vi "find_fish_position.vi"() -> ()   [LabVIEW 2012]
uses:
  labview/find_fish_position.lvlib
  bin/find_fish_position.dll
panel:
  in  "shift":i32=10
  in  "ROI height":i32=256
  in  "ROI width":i32=256
  in  "setROI":bool
  in  "Esize (open)":i32(slide)=4 scale=3.0..10.0
  out "Centroid":cluster{"y":i32, "x":i32}
  out "Image":T1(plugin-control)
  in  "Esize (close)":i32(slide)=4 scale=3.0..10.0
  in  "Threshold":i32(slide)=205 scale=50.0..255.0
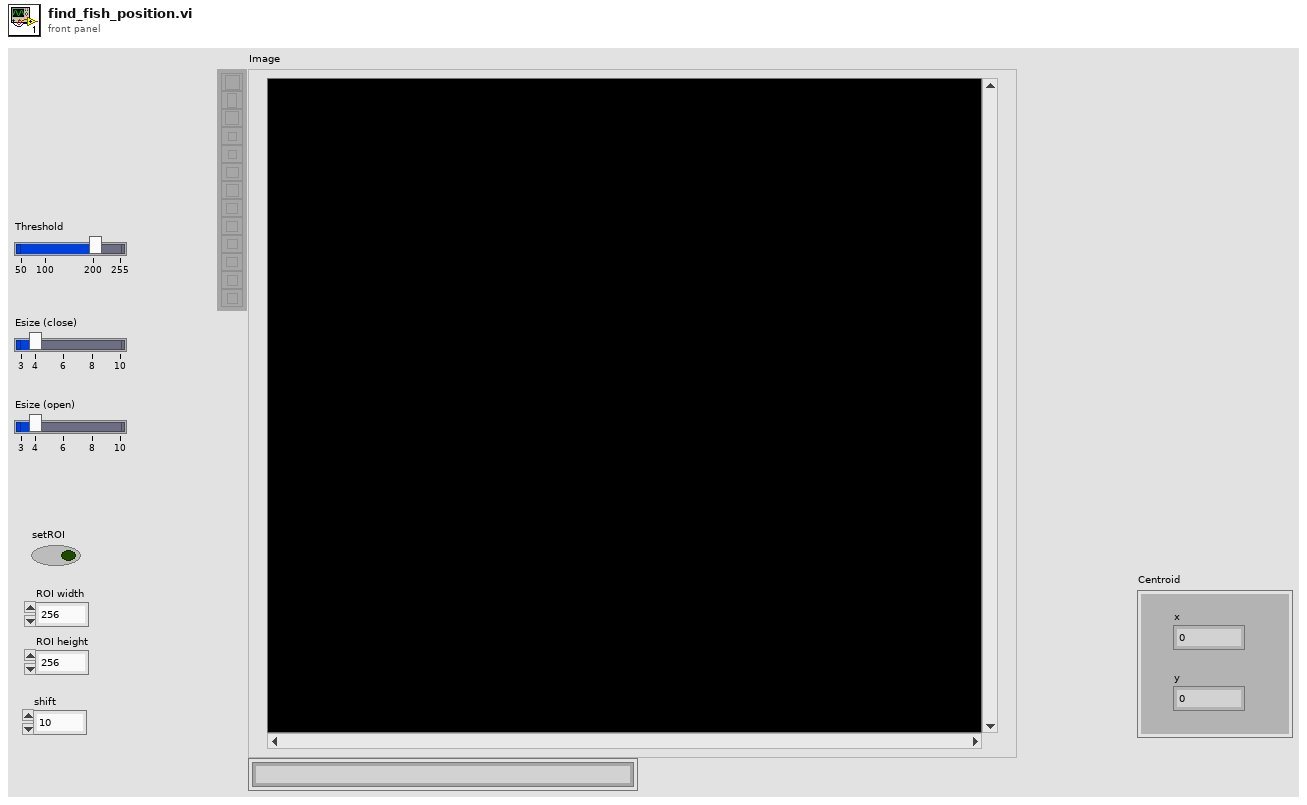
[diagram p1: front panel]
types:
  T1 = typedef "IMAQ Image.ctl" = refnum<image>
  T2 = enum32{"Map Pixel Pointer", "Unmap Pixel Pointer", "Get Pixels Infos"}
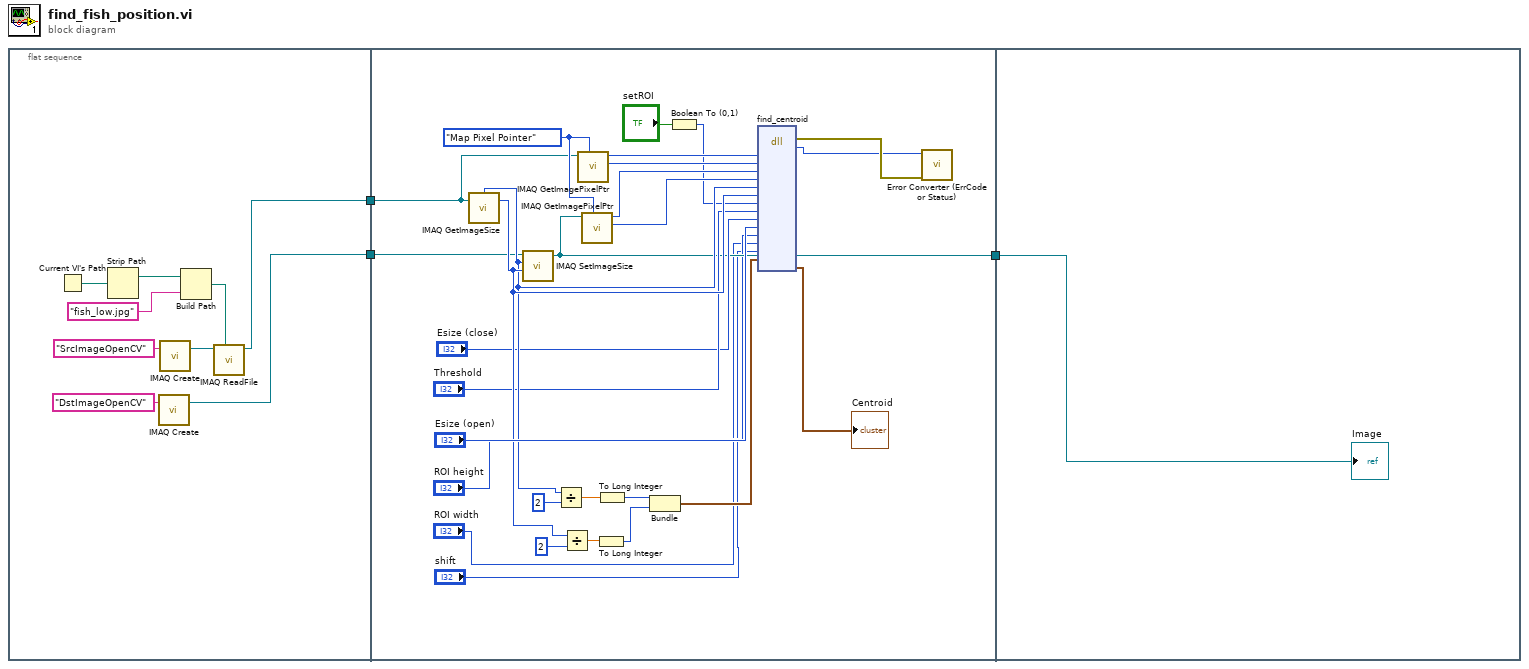
[diagram p0: block diagram]
diagram:
  n1 = flat-sequence {
    tunnel: [w5] -> w3
    tunnel: [w4] -> w2
    tunnel: w3 -> [w25]
    tunnel: w2 -> [w24]
    tunnel: [w23] -> w1
    tunnel: w1 -> [w41]
    frame #0 {
      n2 = Current VI's Path() -> (path=w8:path)
      n3 = Strip Path(path=w8) -> (stripped path=w9:path)  [unwired: 1 out]
      n4 = call "IMAQ Create"("Image Name"="DstImageOpenCV") -> ("New Image"=w4:T1)  [unwired: 4 in, 1 out]
      n5 = call "IMAQ Create"("Image Name"="SrcImageOpenCV") -> ("New Image"=w7:T1)  [unwired: 4 in, 1 out]
      n6 = Build Path(base path=w9, name or relative path="fish_low.jpg") -> (appended path=w6:path)
      n7 = call "IMAQ ReadFile"("File Path"=w6, "Image"=w7) -> ("Image Out"=w5:T1)  [unwired: 5 in, 4 out]
    }
    frame #1 {
      w26 = T2."Map Pixel Pointer" ("Function")
      n8 = call "IMAQ GetImageSize"("Image"=w25) -> ("Y Resolution"=w37:i32, "X Resolution"=w35:i32)  [unwired: 3 in, 1 out]
      n9 = call "IMAQ SetImageSize"("Y Resolution"=w37, "X Resolution"=w35, "Image"=w24) -> ("Image Out"=w23:T1)  [unwired: 2 in, 1 out]
      n10 = Divide(x=w35, y=2) -> (x/y=w20:dbl)
      n11 = Divide(x=w37, y=2) -> (x/y=w18:dbl)
      n12 = call "IMAQ GetImagePixelPtr"("Function"=w26, "Image"=w25) -> ("LineWidth(Pixels)"=w28:i32, "Pixel Pointer out"=w27:u64)  [unwired: 4 in, 4 out]
      n13 = call "IMAQ GetImagePixelPtr"("Function"=w26, "Image"=w23) -> ("LineWidth(Pixels)"=w30:i32, "Pixel Pointer out"=w29:u64)  [unwired: 4 in, 4 out]
      n14 = To Long Integer(number=w18) -> (32bit integer=w17:i32)
      n15 = To Long Integer(number=w20) -> (32bit integer=w19:i32)
      n16 = Bundle(w19, w17) -> (w38:cluster{i32, i32})  [unwired: 1 in]
      n17 = Boolean To (0,1)(Boolean="setROI") -> (0, 1=w21:i16)
      n18 = dll-call lib="C:/Users/quan/workspace/fish tracking dll/bin/find_fish_position.dll" fn="find_centroid"("ImagePtrSrc"=w27, "LineWidthSrc"=w28, "ImagePtrDst"=w29, "LineWidthDst"=w30, "Width"=w35, "Height"=w37, "setROI"=w21, "BinThreshold"="Threshold", "Esize_close"="Esize (close)", "Esize_open"="Esize (open)", "ROI_width"="ROI height", "ROI_height"="ROI width", "shift"="shift", "centroid_in"=w38) -> (error out=w33:errorcluster, "return type"=w13:i32, "Centroid"=→"Centroid":cluster{"y":i32, "x":i32})  [unwired: 18 in, 1 out]
      n19 = call "Error Converter (ErrCode or Status).vi"("error in (no error)"=w33, "error code"=w13) -> ()  [unwired: 9 in, 1 out]
    }
    frame #2 {
      "Image" <- w41
    }
  }
